vi "Task ID.vi"(8 "error in (no error)":errorcluster, 11 "DataProcessor in":refnum<class "DataProcessor.lvclass">) -> (0 "error out":errorcluster, 2 "Task ID":string, 3 "DataProcessor out":refnum<class "DataProcessor.lvclass">)   [LabVIEW 2020, in "Volatus.lvlib" / "DataProcessor.lvclass"]
uses:
  DataProcessor.lvclass
  C:/dev/lv20CE/relink/lv-volatus/Volatus/DataHandlerTask/DataHandlerTask.lvclass
  Volatus/DataHandlerTask/DataHandlerTask.lvclass/DataHandlerTask.ctl
  DataProcessor.lvclass/DataProcessor.ctl
  Volatus/DataHandlerTask/DataHandlerTask.lvclass
  C:/dev/lv20CE/relink/lv-volatus/Volatus/Task/Task.lvclass
  C:/Program Files (x86)/National Instruments/LabVIEW 2020/vi.lib/ActorFramework/Actor/Actor.lvclass
  C:/dev/lv20CE/relink/lv-volatus/Volatus/TaskStateHandler/TaskStateHandler.lvclass
  C:/dev/lv20CE/relink/lv-volatus/Volatus/VectoMessageHandler/VectoMessageHandler.lvclass
  C:/dev/lv20CE/relink/lv-volatus/Volatus/API Provider/API Provider.lvclass
  C:/dev/lv20CE/relink/lv-volatus/Volatus/DataHandler/DataHandler.lvclass
  C:/dev/lv20CE/relink/lv-volatus/VolatusDataProcessing/DataProcessor/DataProcessor.lvclass
  C:/dev/lv20CE/relink/lv-volatus/Volatus/AbortHandler/AbortHandler.lvclass
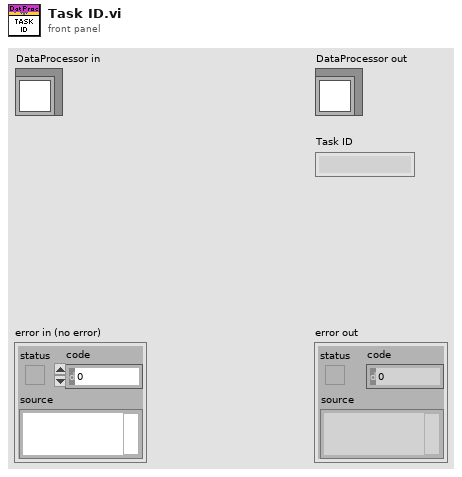
[diagram p1: front panel]
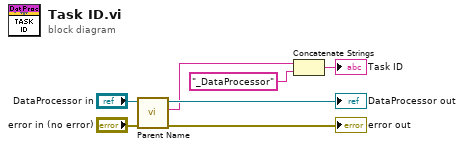
[diagram p0: block diagram]
diagram:
  n1 = call "Parent Name.vi"("error in (no error)"="error in (no error)", "DataHandlerTask in"="DataProcessor in") -> ("error out"=→"error out":errorcluster, "Parent Name"=w3:string, "DataHandlerTask out"=→"DataProcessor out":refnum<class "DataProcessor.lvclass">)  [unwired: 7 in]
  n2 = Concatenate Strings(w3, "_DataProcessor" ("Task ID")) -> (→"Task ID":string)
